vi "set_new_position.vi"(8 "error in (no error)":errorcluster, 10 "set_pos":dbl[](array[numeric]), 11 "smc100 in":refnum<class "smc100.lvclass">) -> (0 "error out":errorcluster, 3 "smc100 out":refnum<class "smc100.lvclass">)   [LabVIEW 2019, in "smc100.lvlib" / "smc100.lvclass"]
uses:
  smc100.lvclass
  smc100.lvclass/smc100.ctl
  Read VISA Handle.vi
  smc100.lvlib
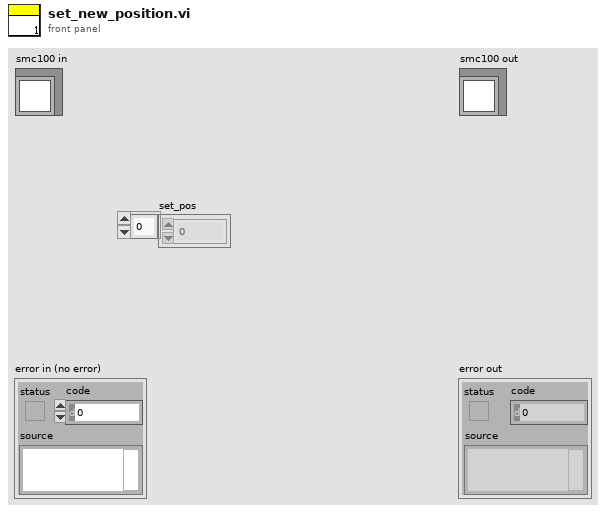
[diagram p1: front panel]
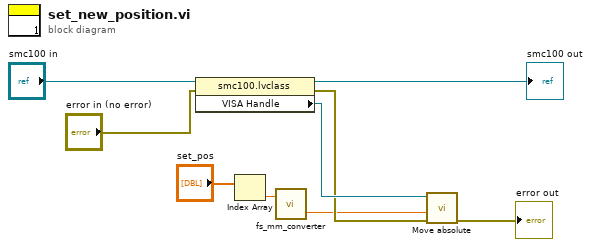
[diagram p0: block diagram]
diagram:
  n1 = property class="smc100.lvclass"(reference="smc100 in", error in="error in (no error)") -> (reference out=→"smc100 out":refnum<class "smc100.lvclass">, error out=w7:errorcluster, "VISA Handle"=w8:refnum<visa-resource-name>)
  n2 = Index Array(array="set_pos") -> (element=w2:dbl)  [unwired: 1 in]
  n3 = call "fs_mm_converter.vi"("fs in"=w2) -> ("mm out"=w1:dbl)  [unwired: 1 in, 1 out]
  n4 = call <userlib>:"Move absolute.vi"("error in"=w7, "New target position (units)"=w1, "VISA Handle in"=w8) -> ("error out"=→"error out":errorcluster)  [unwired: 3 in, 3 out]
